vi "check_timeout.vi"(8 "error in (no error)":errorcluster, 11 "ExperimentVariables in":refnum<class "ExperimentVariables.lvclass">) -> (0 "error out":errorcluster, 2 "timeout elapsed?":bool, 3 "ExperimentVariables out":refnum<class "ExperimentVariables.lvclass">)   [LabVIEW 2013, in "ExperimentVariables.lvclass"]
uses:
  ExperimentVariables.lvclass
  ExperimentVariables.lvclass/ExperimentVariables.ctl
  Experiment/Globals.vi
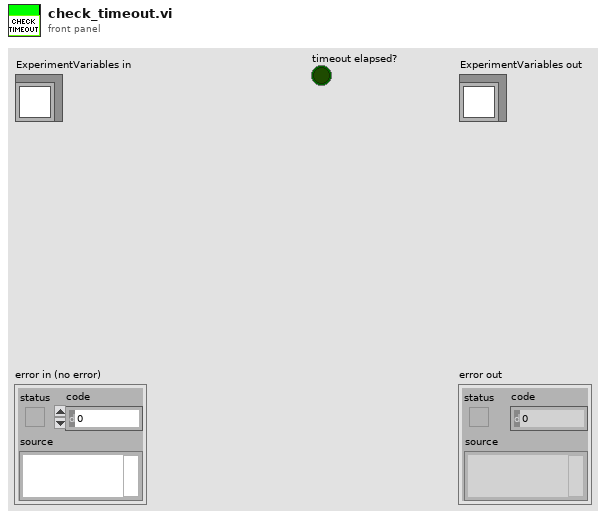
[diagram p1: front panel]
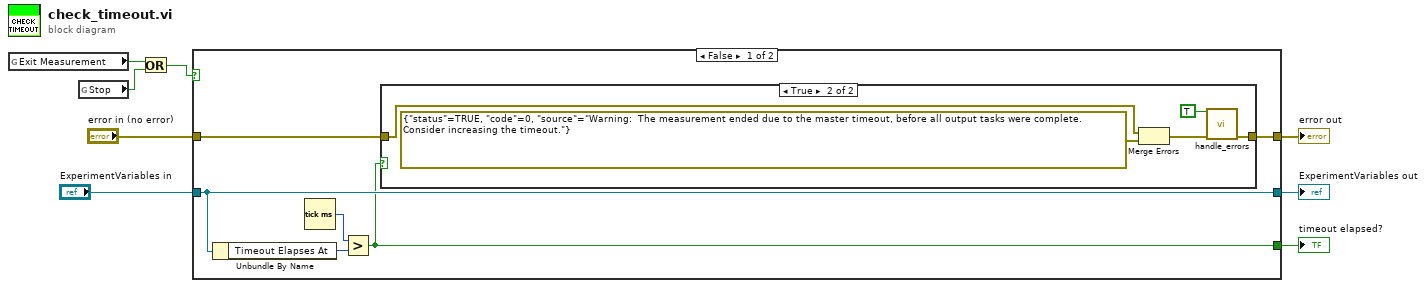
[diagram p0: block diagram]
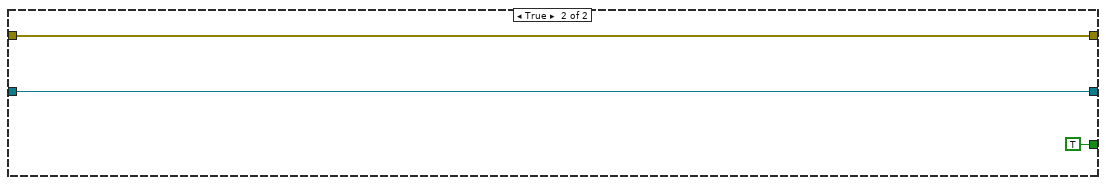
[diagram p3: hidden frame]
diagram:
  n1 = global read "Globals.vi" "Exit Measurement"() -> (w3:bool)
  n2 = global read "Globals.vi" "Stop"() -> (w2:bool)
  n3 = Or(x=w3, y=w2) -> (x .or. y?=w1:bool)
  n4 = case shown="False" w1 {
    tunnel: [w11 w22] -> w5
    tunnel: [w14 w23] -> w7
    tunnel: "ExperimentVariables in" -> [w14 w23]
    tunnel: [w10 TRUE] -> w6
    tunnel: "error in (no error)" -> [w9 w22]
    frame False {
      n5 = Unbundle By Name(w14) -> ("Timeout Elapses At"=w12:u32)
      n6 = Tick Count (ms)() -> (millisecond timer value=w13:u32)
      n7 = Greater?(x=w13, y=w12) -> (0:w10:bool)
      n8 = case shown="True" w10 {
        tunnel: [w15 w18] -> w11
        tunnel: w9 -> [w15 w17]
        frame False {
        }
        frame True {
          n9 = Merge Errors(w17, errorcluster {"status"=TRUE, "code"=0, "source"="Warning:  The measurement ended due to the master timeout, before all output tasks were complete.  Consider increasing the timeout."} ("error constant")) -> (w19:errorcluster)
          n10 = call "handle_errors.vi"("Exit Operation"=TRUE ("Exit Measurement"), "error in (no error)"=w19) -> ("error out"=w18:errorcluster)  [unwired: 13 in]
        }
      }
    }
    frame True {
    }
  }
  "error out" <- w5
  "ExperimentVariables out" <- w7
  "timeout elapsed?" <- w6
